vi "Clear Buffer.vi"(8 "error in":errorcluster, 11 "Refnum in":T1) -> (0 "error out":errorcluster, 3 "FPGA VI Reference Out":T1)   [LabVIEW 2015, in "Open Path CRD.lvclass"]
doc: "Pause the digitization and clear any samples that may be in the buffer. IMPORTANT: Restart the digitizer AFTER this VI is called!!!"
uses:
  Open Path CRD.lvclass
  Open Path FPGA Ref.ctl
  <vilib>/Utility/error.llb/Error Cluster From Error Code.vi
  <vilib>/rvi/errors/niLvFpgaAdjustHostInterfaceError.vi
  <vilib>/rvi/interface/nirviReadWriteControl/nirviReadWriteControl.xnode
  FPGA Bitfiles/Handix_OpenPathCRD.lvbitx
  <vilib>/rvi/interface/nirviMethod/nirviMethod.xnode
  <vilib>/rvi/errors/niLvFpgaMergeErrorWithErrorCode.vi
  <vilib>/FPGAPlugInAG/sbRIO-9637/niLvFpga_ReadFifo_sbRIO-9637.vi
  NiFpgaLv.dll
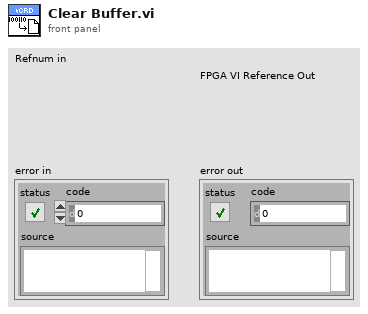
[diagram p1: front panel]
types:
  T1 = typedef "Open Path CRD.lvclass/Open Path FPGA Ref.ctl" = refnum<k20>
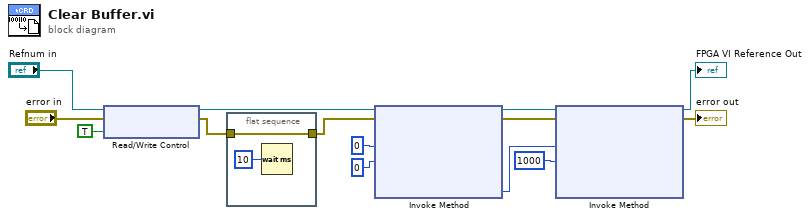
[diagram p0: block diagram]
diagram:
  n1 = xnode "Read/Write Control"("FPGA VI Reference In"="Refnum in", "error in"="error in", "Pause Digitizer"=TRUE) -> ("FPGA VI Reference Out"=w1:T1, "error out"=w3:errorcluster)
  n2 = flat-sequence {
    tunnel: w3 -> [w15]
    tunnel: [w15] -> w2
    frame #0 {
      n3 = Wait (ms)(milliseconds to wait=u32 10) -> ()  [unwired: 1 out]
    }
  }
  n4 = xnode "Invoke Method"("FPGA VI Reference In"=w1, "error in"=w2, "Number of Elements"=u32 0, "Timeout (ms)"=0) -> ("FPGA VI Reference Out"=w8:T1, "error out"=w5:errorcluster, "Elements Remaining"=w7:u32)  [unwired: 1 out]
  n5 = xnode "Invoke Method"("FPGA VI Reference In"=w8, "error in"=w5, "Number of Elements"=w7, "Timeout (ms)"=1000) -> ("FPGA VI Reference Out"=→"FPGA VI Reference Out":T1, "error out"=→"error out":errorcluster)  [unwired: 2 out]
